vi "Find Register Offset.vi"(8 "error in (no error)":errorcluster, 10 "register name":string, 11 "session in":u32) -> (0 "error out":errorcluster, 2 "resource offset":u32, 3 "session out":u32)   [LabVIEW 2018, in "Scalar IO Operations.lvlib"]
uses:
  Scalar IO Operations.lvlib
  TypeDefs/Register Data Store.ctl
  NiFpga.dll
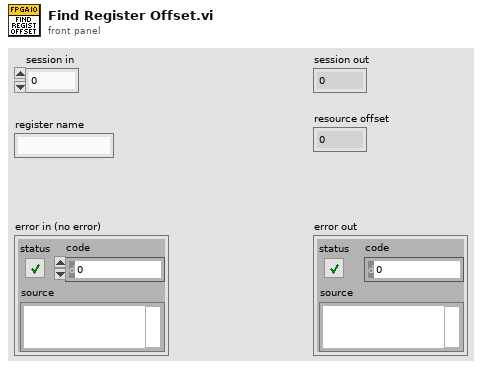
[diagram p1: front panel]
types:
  T1 = typedef "Scalar IO Operations.lvlib/Register Data Store.ctl" = cluster{"Register Names":string[], "Register Offset":u32[]}
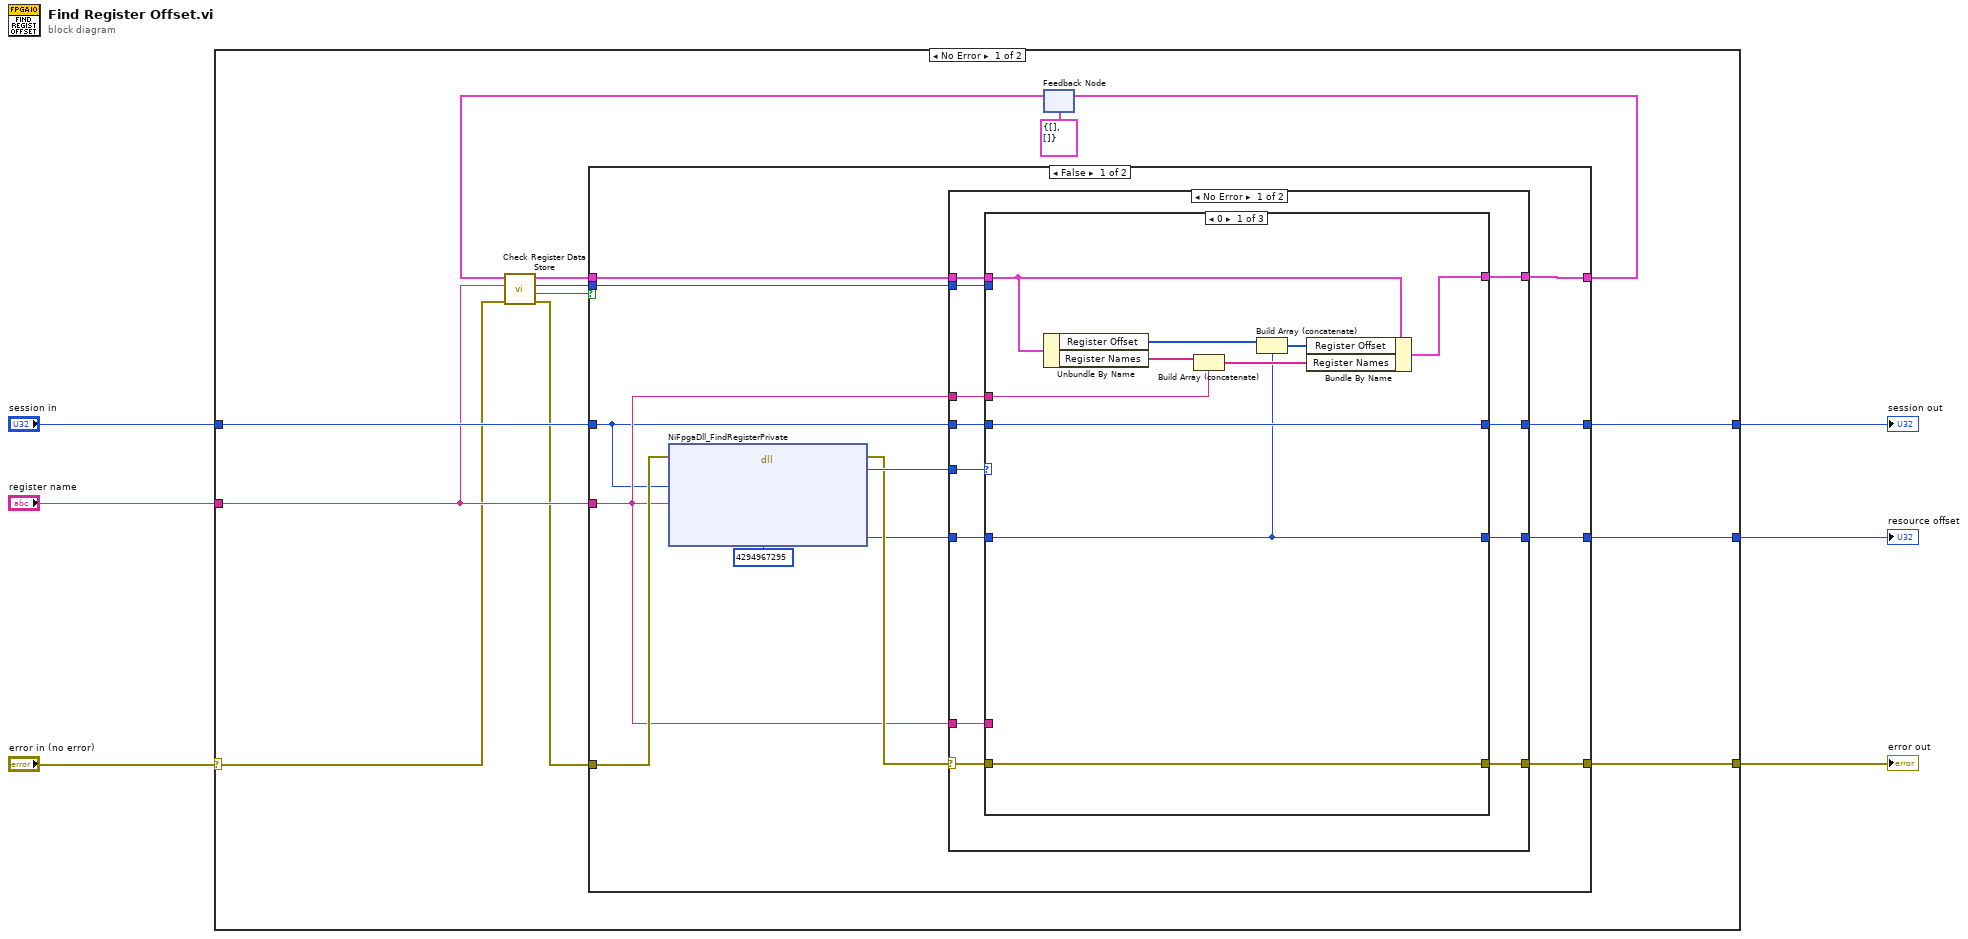
[diagram p0: block diagram]
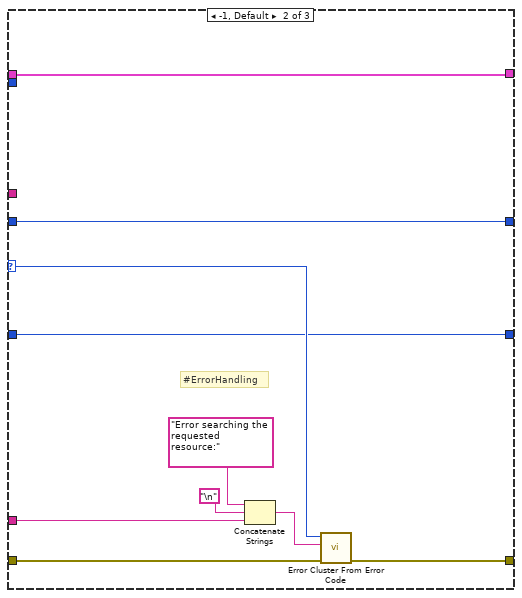
[diagram p2: hidden frame]
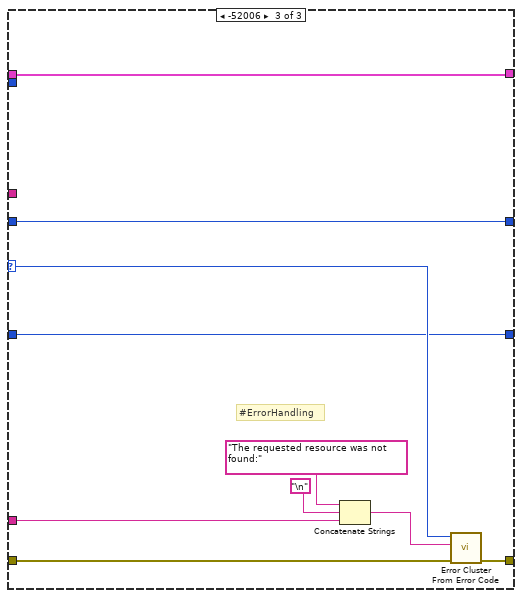
[diagram p3: hidden frame]
diagram:
  n1 = case shown="No Error" "error in (no error)" {
    selector: "error in (no error)" -> [w9 w84]
    tunnel: [w18 w84] -> w3
    tunnel: "register name" -> [w13 _]
    tunnel: "session in" -> [w19 w83]
    tunnel: [w17 w83] -> w4
    tunnel: [w16 _] -> w2
    frame No Error {
      n2 = feedback #1(T1 {"Register Names"=[], "Register Offset"=[]}) -> (w14:T1)
      n3 = call "Check Register Data Store.vi"("error in (no error)"=w9, "register name"=w13, "register data store in"=w14) -> ("error IO"=w8:errorcluster, "Found"=w7:bool, "register offset"=w11:u32, "register data store out"=w12:T1)  [unwired: 5 in]
      n4 = case shown="False" w7 {
        tunnel: w8 -> [w31 w81]
        tunnel: w19 -> [w22 w82]
        tunnel: [w20 w79] -> w16
        tunnel: [w29 w81] -> w18
        tunnel: [w21 w82] -> w17
        tunnel: w13 -> [w25 _]
        tunnel: w12 -> [w27 w80]
        tunnel: w11 -> [w26 w79]
        tunnel: [w23 w80] -> w10
        frame False {
          n5 = dll-call lib="NiFpga.*" fn="NiFpgaDll_FindRegisterPrivate"(error in=w31, "session"=w22, "registerName"=w25, "expectedResourceType"=u32 4294967295) -> (error out=w28:errorcluster, "status"=w30:i32, "resourceOffset"=w24:u32)  [unwired: 6 in, 1 out]
          n6 = case shown="No Error" w28 {
            selector: w28 -> [w41 w78]
            tunnel: w30 -> [w44 _]
            tunnel: [w43 w78] -> w29
            tunnel: w25 -> [w42 _]
            tunnel: w27 -> [w40 w75]
            tunnel: w26 -> [w39 _]
            tunnel: w25 -> [w38 _]
            tunnel: w24 -> [w37 w76]
            tunnel: [w36 w75] -> w23
            tunnel: w22 -> [w35 w77]
            tunnel: [w34 w77] -> w21
            tunnel: [w33 w76] -> w20
            frame No Error {
              n7 = case shown="0" w44 {
                selector: w44 -> [_ w62 w73]
                tunnel: [w54 w63 w74] -> w43
                tunnel: w42 -> [_ w58 w70]
                tunnel: w41 -> [w54 w64 w68]
                tunnel: w40 -> [w48 w57 w66]
                tunnel: w39 -> [_ _ _]
                tunnel: w38 -> [w51 _ _]
                tunnel: w37 -> [w45 w55 w65]
                tunnel: [w47 w57 w66] -> w36
                tunnel: w35 -> [w46 w56 w67]
                tunnel: [w46 w56 w67] -> w34
                tunnel: [w45 w55 w65] -> w33
                frame 0 {
                  n8 = Unbundle By Name(w48) -> ("Register Offset"=w53:u32[], "Register Names"=w52:string[])
                  n9 = Build Array (concatenate)(w52, w51) -> (w49:string[])
                  n10 = Build Array (concatenate)(w53, w45) -> (w50:u32[])
                  n11 = Bundle By Name(cluster=w48, "Register Offset"=w50, "Register Names"=w49) -> (w47:T1)
                }
                frame -1, Default {
                  # "#ErrorHandling"
                  n12 = Concatenate Strings("Error searching the requested resource:" ("error message (\"\")"), "\n", w58) -> (w59:string)
                  n13 = call <vilib>:"Error Cluster From Error Code.vi"("error in (no error)"=w64, "error message (\"\")"=w59, "error code (0)"=w62) -> ("error out"=w63:errorcluster)  [unwired: 6 in]
                }
                frame -52006 {
                  # "#ErrorHandling"
                  n14 = Concatenate Strings("The requested resource was not found:" ("error message (\"\")"), "\n", w70) -> (w69:string)
                  n15 = call <vilib>:"Error Cluster From Error Code.vi"("error in (no error)"=w68, "error message (\"\")"=w69, "error code (0)"=w73) -> ("error out"=w74:errorcluster)  [unwired: 6 in]
                }
              }
            }
            frame Error {
            }
          }
        }
        frame True {
        }
      }
      n16 = feedback-in #1(w10) -> ()
    }
    frame Error {
    }
  }
  "session out" <- w4
  "error out" <- w3
  "resource offset" <- w2
